vi "Initialize.vi"(8 "error in (no error)":errorcluster, 11 "Settings Editor in":refnum<class "Settings Editor.lvclass">) -> (0 "error out":errorcluster, 3 "Settings Editor out":refnum<class "Settings Editor.lvclass">)   [LabVIEW 2017, in "DSF Core.lvlib" / "Settings Editor.lvclass"]
uses:
  Settings Editor.lvclass
  C:/Git/DSF/Core/Classes/User Interface/User Interface.lvclass
  Settings Editor.lvclass/Settings Editor.ctl
  User Interface.vi
  User Interface.lvclass
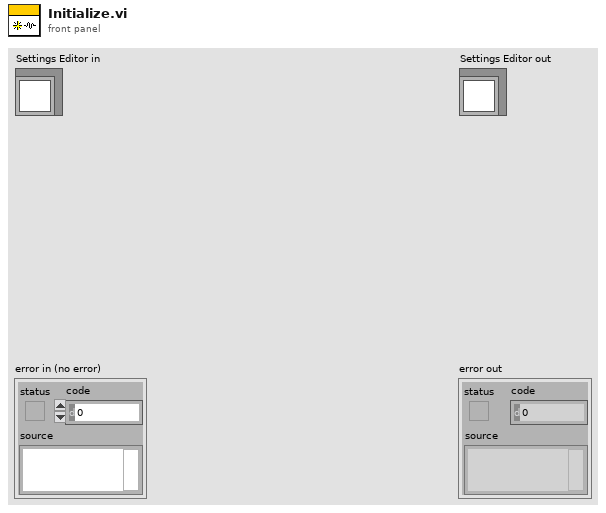
[diagram p1: front panel]
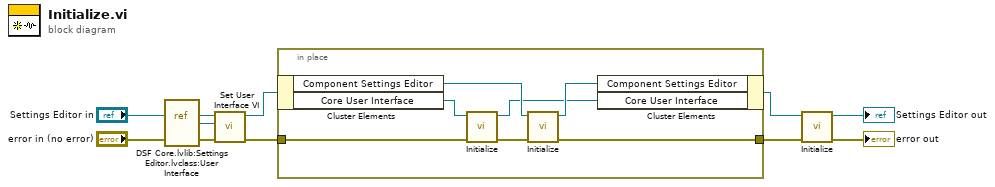
[diagram p0: block diagram]
diagram:
  n1 = vi-ref "DSF Core.lvlib:Settings Editor.lvclass:User Interface.vi"() -> (w7:refnum<vi>)
  n2 = call "Set User Interface VI.vi"("error in (no error)"="error in (no error)", "vi"=w7, "User Interface in"="Settings Editor in") -> ("error out"=w3:errorcluster, "User Interface out"=w4:refnum<class "Settings Editor.lvclass">)  [unwired: 7 in]
  n3 = in-place {
    in-place-border: w3 -> [w16]
    in-place-border: [w12] -> w2
    n4 = in-place-cluster #1(w4) -> ("Component Settings Editor"=w13:refnum<class "User Interface.lvclass">, "Core User Interface"=w15:refnum<class "User Interface.lvclass">)
    n5 = call-dynamic "Initialize.vi"("error in (no error)"=w16, "User Interface in"=w15) -> ("error out"=w14:errorcluster, "User Interface out"=w10:refnum<class "User Interface.lvclass">)  [unwired: 8 in]
    n6 = call-dynamic "Initialize.vi"("error in (no error)"=w14, "User Interface in"=w13) -> ("error out"=w12:errorcluster, "User Interface out"=w11:refnum<class "User Interface.lvclass">)  [unwired: 8 in]
    n7 = in-place-cluster #1("Component Settings Editor"=w11, "Core User Interface"=w10) -> (w1:refnum<class "Settings Editor.lvclass">)
  }
  n8 = call-parent "Initialize.vi"("error in (no error)"=w2, "User Interface in"=w1) -> ("error out"=→"error out":errorcluster, "User Interface out"=→"Settings Editor out":refnum<class "Settings Editor.lvclass">)  [unwired: 8 in]
